vi "mules_close_window.vi"(8 "error in (no error)":errorcluster, 11 "IpszWindowName":string="C:\\Program Files (x86)\\National Instruments\\LabVIEW 2013\\user.lib\\cassani" caption="WindowName") -> (0 "sortie d'erreur":errorcluster caption="error out")   [LabVIEW 2013]
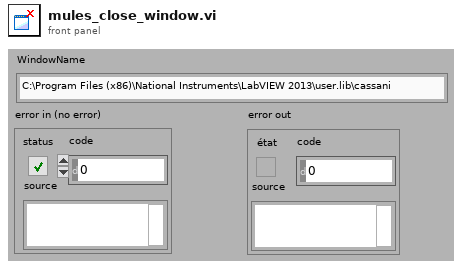
[diagram p1: front panel]
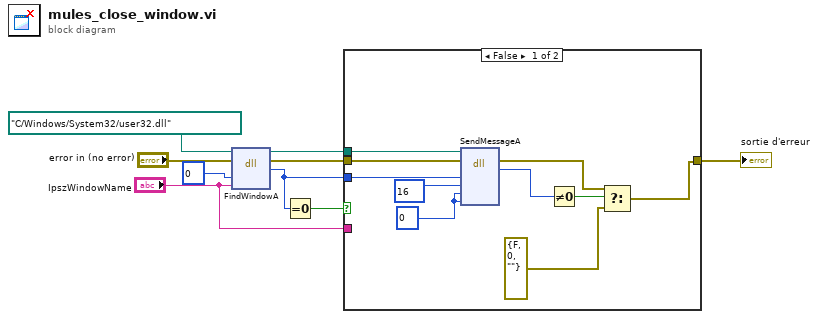
[diagram p0: block diagram]
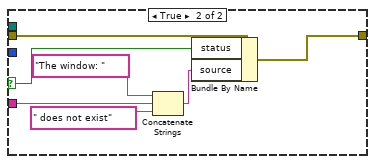
[diagram p2: hidden frame]
diagram:
  n1 = dll-call lib="?" fn="FindWindowA" label="FindWindow"(path in=path "C:/Windows/System32/user32.dll", error in="error in (no error)", "IpszClassName"=0, "IpszWindowName"="IpszWindowName") -> (path out=w1:path, error out=w6:errorcluster, "type de retour"=w4:u32)  [unwired: 3 in]
  n2 = Equal To 0?(x=w4) -> (x = 0?=w7:bool)
  n3 = case shown="False" w7 {
    selector: w7 -> [_ w25]
    tunnel: w6 -> [w18 w26]
    tunnel: [w11 w20] -> w8
    tunnel: "IpszWindowName" -> [_ w22]
    tunnel: w4 -> [w16 _]
    tunnel: w1 -> [w10 _]
    frame False {
      w17 = u32 0 ("IParam")
      n4 = dll-call lib="C:/Windows/System32/user32.dll" fn="SendMessageA" label="SendMessage"(path in=w10, error in=w18, "hWnd"=w16, "uMsg"=u32 16 ("wParam"), "wParam"=w17, "IParam"=w17) -> (error out=w12:errorcluster, "type de retour"=w15:u32)  [unwired: 5 in, 1 out]
      n5 = Not Equal To 0?(x=w15) -> (x != 0?=w14:bool)
      n6 = Select(t=w12, s=w14, f=errorcluster {"status"=FALSE, "code"=0, "source"=""} ("sortie d'erreur")) -> (s? t:f=w11:errorcluster)
    }
    frame True {
      n7 = Concatenate Strings("The window: " ("source"), w22, " does not exist" ("source")) -> (w24:string)
      n8 = Bundle By Name(cluster=w26, "status"=w25, "source"=w24) -> (w20:errorcluster)
    }
  }
  "sortie d'erreur" <- w8
